vi "read-block.vi"(11 "Byte Stream File in":refnum<file>) -> (2 "Array":dbl[](array[numeric]), 3 "Byte Stream File out":refnum<file>)   [LabVIEW 2011]
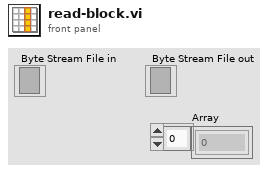
[diagram p1: front panel]
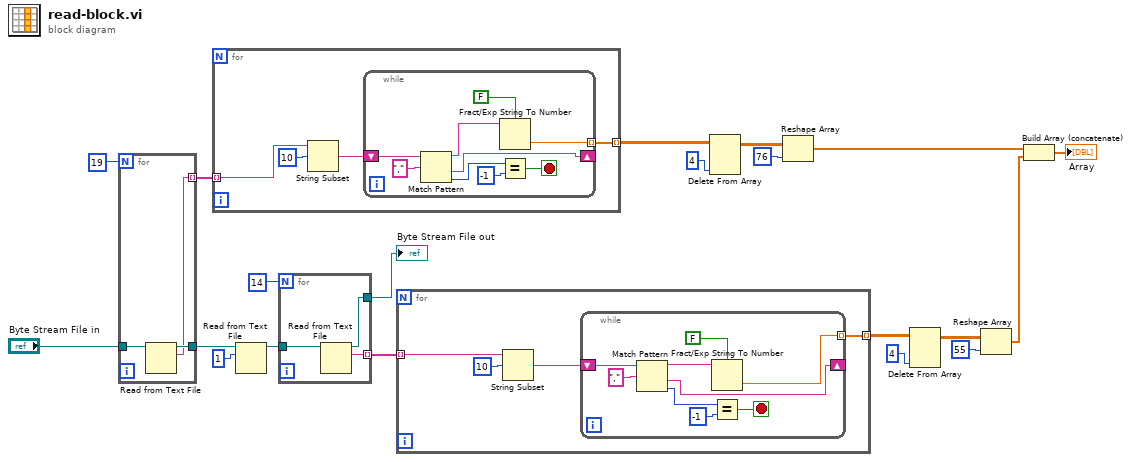
[diagram p0: block diagram]
diagram:
  n1 = for {
    N: 19 ("Numeric") -> [_]
    tunnel: "Byte Stream File in" -> [w23]
    tunnel: [w22] -> w2
    tunnel: [w21] -> w4 mode=indexing
    n2 = Read from Text File(file (use dialog)=w23) -> (refnum out=w22:refnum<file>, text=w21:string)  [unwired: 3 in, 2 out]
  }
  n3 = for {
    tunnel: w4 -> [w25] mode=indexing
    tunnel: [w26] -> w5 mode=indexing
    n4 = String Subset(string=w25, offset (0)=10) -> (substring=w24:string)  [unwired: 1 in]
    n5 = while {
      shift-right: [w34] -> _
      shift-left: w24 -> [w36]
      tunnel: [w33] -> w26 mode=indexing
      stop <- w30 stop-if-true
      n6 = Match Pattern(string=w36, regular expression=",") -> (before substring=w35:string, after substring=w34:string, offset past match=w32:i32)  [unwired: 1 in, 1 out]
      n7 = Fract/Exp String To Number(use system decimal point (T)=FALSE, string=w35) -> (number=w33:dbl)  [unwired: 2 in, 1 out]
      n8 = Equal?(x=w32, y=-1) -> (x = y?=w30:bool)
    }
  }
  n9 = Read from Text File(file (use dialog)=w2, count=1) -> (refnum out=w8:refnum<file>)  [unwired: 2 in, 3 out]
  n10 = for {
    N: 14 ("Numeric") -> [_]
    tunnel: w8 -> [w39]
    tunnel: [w38] -> w20
    tunnel: [w37] -> w10 mode=indexing
    n11 = Read from Text File(file (use dialog)=w39) -> (refnum out=w38:refnum<file>, text=w37:string)  [unwired: 3 in, 2 out]
  }
  "Byte Stream File out" <- w20
  n12 = for {
    tunnel: w10 -> [w41] mode=indexing
    tunnel: [w42] -> w11 mode=indexing
    n13 = String Subset(string=w41, offset (0)=10) -> (substring=w40:string)  [unwired: 1 in]
    n14 = while {
      shift-right: [w50] -> _
      shift-left: w40 -> [w52]
      tunnel: [w49] -> w42 mode=indexing
      stop <- w46 stop-if-true
      n15 = Match Pattern(string=w52, regular expression=",") -> (before substring=w51:string, after substring=w50:string, offset past match=w48:i32)  [unwired: 1 in, 1 out]
      n16 = Fract/Exp String To Number(use system decimal point (T)=FALSE, string=w51) -> (number=w49:dbl)  [unwired: 2 in, 1 out]
      n17 = Equal?(x=w48, y=-1) -> (x = y?=w46:bool)
    }
  }
  n18 = Delete From Array(array=w5, index (col)=4 ("disabled index (col)")) -> (array with subset deleted=w13:dbl[][])  [unwired: 2 in, 1 out]
  n19 = Reshape Array(w13, 76 ("dimension size")) -> (w17:dbl[])
  n20 = Delete From Array(array=w11, index (col)=4 ("disabled index (col)")) -> (array with subset deleted=w16:dbl[][])  [unwired: 2 in, 1 out]
  n21 = Reshape Array(w16, 55 ("dimension size")) -> (w18:dbl[])
  n22 = Build Array (concatenate)(w17, w18) -> (→"Array":dbl[])
